vi "字符串操作函数（一）.vi"() -> ()   [LabVIEW 2010]
panel:
  out "全部小写":string
  out "全部大写":string
  out "部分字符串":string
  out "连接后的字符串":string="LabVIEW\rString\rOperateFunction"
  out "字符串长度":i32
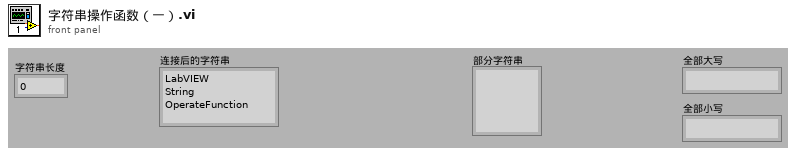
[diagram p1: front panel]
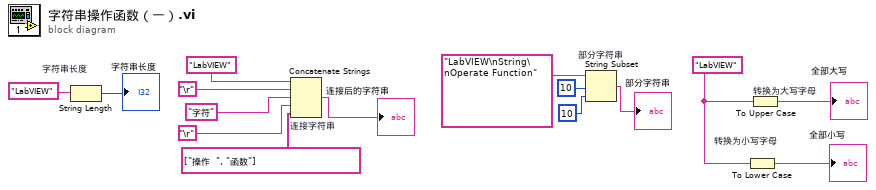
[diagram p0: block diagram]
diagram:
  w1 = "LabVIEW"
  n1 = String Length "字符串长度"(string="LabVIEW") -> (length=→"字符串长度":i32)
  n2 = Concatenate Strings "连接字符串"("LabVIEW", "\r", "字符", "\r", string[] ["操作  ", "函数"]) -> (→"连接后的字符串":string)
  n3 = String Subset "部分字符串"(string="LabVIEW\nString\nOperate Function", offset (0)=10, length (rest)=10) -> (substring=→"部分字符串":string)
  n4 = To Lower Case "转换为小写字母"(string=w1) -> (all lower case string=→"全部小写":string)
  n5 = To Upper Case "转换为大写字母"(1:w1) -> (0:→"全部大写":string)
